vi "WriteCsv.vi"(1 "相对路径":string, 2 "1D data":string[](array[string]) caption="一维数据", 3 "2D data":string[][](array[string]) caption="二维数据", 4 "路径":path) -> (0 "布尔":bool)   [LabVIEW 2018]
uses:
  <vilib>/Utility/file.llb/Write Delimited Spreadsheet (string).vi
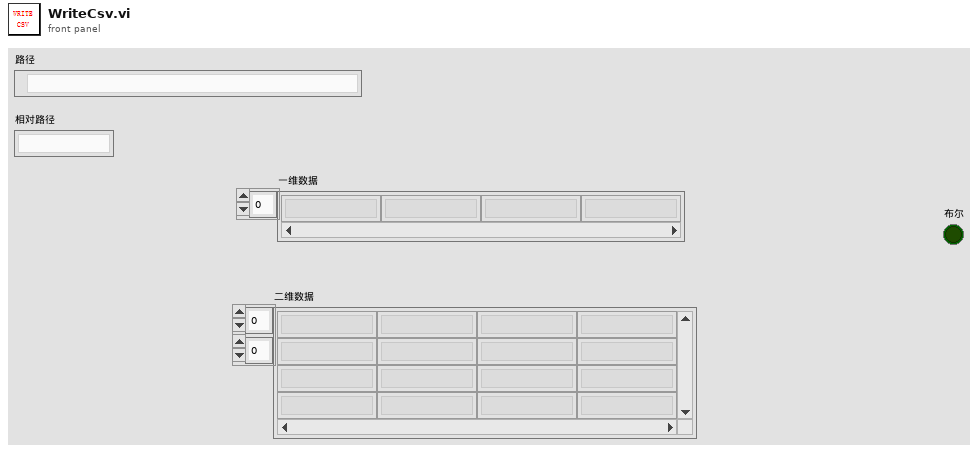
[diagram p1: front panel]
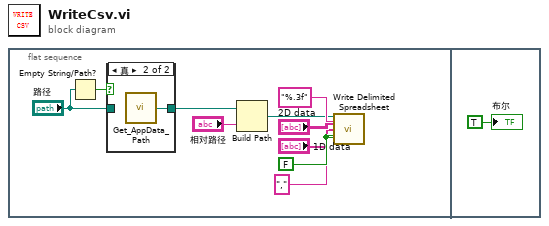
[diagram p0: block diagram]
diagram:
  n1 = flat-sequence {
    frame #0 {
      w4 = FALSE ("append to file? (new file:F)")
      n2 = Empty String/Path?(string/path="路径") -> (empty?=w10:bool)
      n3 = case shown="真" w10 {
        tunnel: "路径" -> [w11 _]
        tunnel: [w11 w12] -> w7
        frame False {
        }
        frame True {
          n4 = call "Get_AppData_Path.vi"() -> ("path"=w12:path)  [unwired: 1 in]
        }
      }
      n5 = Build Path(base path=w7, name or relative path="相对路径") -> (appended path=w5:path)
      n6 = call-poly <vilib>:"Write Delimited Spreadsheet.vi"("file path (dialog if empty)"=w5, "format (%s)"="%.3f" ("format (%.3f)"), "2D data"="2D data", "1D data"="1D data", "append to file? (new file:F)"=w4, "transpose? (no:F)"=w4, "delimiter (\\t)"="," ("delimiter (\\t)")) -> ()  [unwired: 7 in, 2 out]
    }
    frame #1 {
      "布尔" <- TRUE ("布尔")
    }
  }
